vi "Vector to Scalar Array.vi"(1 "Three axis vector":dbl[][](array[numeric])) -> (0 "Total field":dbl[](array[numeric]))   [LabVIEW 2010]
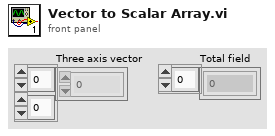
[diagram p1: front panel]
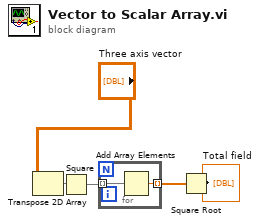
[diagram p0: block diagram]
diagram:
  n1 = Transpose 2D Array(2D array="Three axis vector") -> (transposed array=w4:dbl[][])
  n2 = Square(x=w4) -> (x^2=w1:dbl[][])
  n3 = for {
    tunnel: w1 -> [w7] mode=indexing
    tunnel: [w6] -> w2 mode=indexing
    n4 = Add Array Elements(numeric array=w7) -> (sum=w6:dbl)
  }
  n5 = Square Root(x=w2) -> (sqrt(x)=→"Total field":dbl[])
